vi "Periodic Tasks.vi"(8 "error in":errorcluster) -> ()   [LabVIEW 2015]
doc: "This VI runs in parallel to other tasks. It can contain as many user-defined periodic loops as you need. These can carry out PID or other sorts of timed response."
uses:
  <vilib>/Rock Robotics/WPI/Utilities/WPI_GetSetVariantRefNum.vi
  Robot Global Data.vi
  <vilib>/Rock Robotics/Network Tables/SD Write Number.vi
  <vilib>/Rock Robotics/Network Tables/SD Write Boolean.vi
  <vilib>/Rock Robotics/Network Tables/NT Read Numeric Array.vi
  <vilib>/Rock Robotics/Network Tables/SD Write Numeric Array.vi
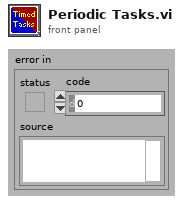
[diagram p1: front panel]
types:
  T1 = typedef "WPI_JoystickDevRef.ctl" = cluster{"Device":T2}
  T2 = typedef "WPI_JoystickDeviceEnum.ctl" = enum16{"USB 0", "USB 1", "USB 2", "USB 3", "USB 4", "USB 5"}
  T3 = cluster{"Axes[0]":dbl, "Axes[1]":dbl, "Axes[2]":dbl, "Axes[3]":dbl, "Axes[4]":dbl, "Axes[5]":dbl, "Axes[6]":dbl, "Axes[7]":dbl, "Axes[8]":dbl}
  T4 = cluster{"Buttons[0]":bool, "Buttons[1]":bool, "Buttons[2]":bool, "Buttons[3]":bool, "Buttons[4]":bool, "Buttons[5]":bool, "Buttons[6]":bool, "Buttons[7]":bool, "Buttons[8]":bool}
  T5 = typedef "WPI_EncoderDevRef.ctl" = cluster{"DevStatus":errorcluster, "EncoderIndex":T6, "CounterIndex":T7, "DistancePerCount":dbl, "Decoding Type":T8}
  T6 = typedef "FPGA_EncoderIdx.ctl" = enum8{"Enc 0", "Enc 1", "Enc 2", "Enc 3", "Enc 4", "Enc 5", "Enc 6", "Enc 7", "Invalid"}
  T7 = typedef "FPGA_CounterCtrSystemIndex.ctl" = enum8{"Ctr 0", "Ctr 1", "Ctr 2", "Ctr 3", "Ctr 4", "Ctr 5", "Ctr 6", "Ctr 7", "Invalid"}
  T8 = typedef "WPI_EncoderType.ctl" = enum16{"1x", "2x", "4x"}
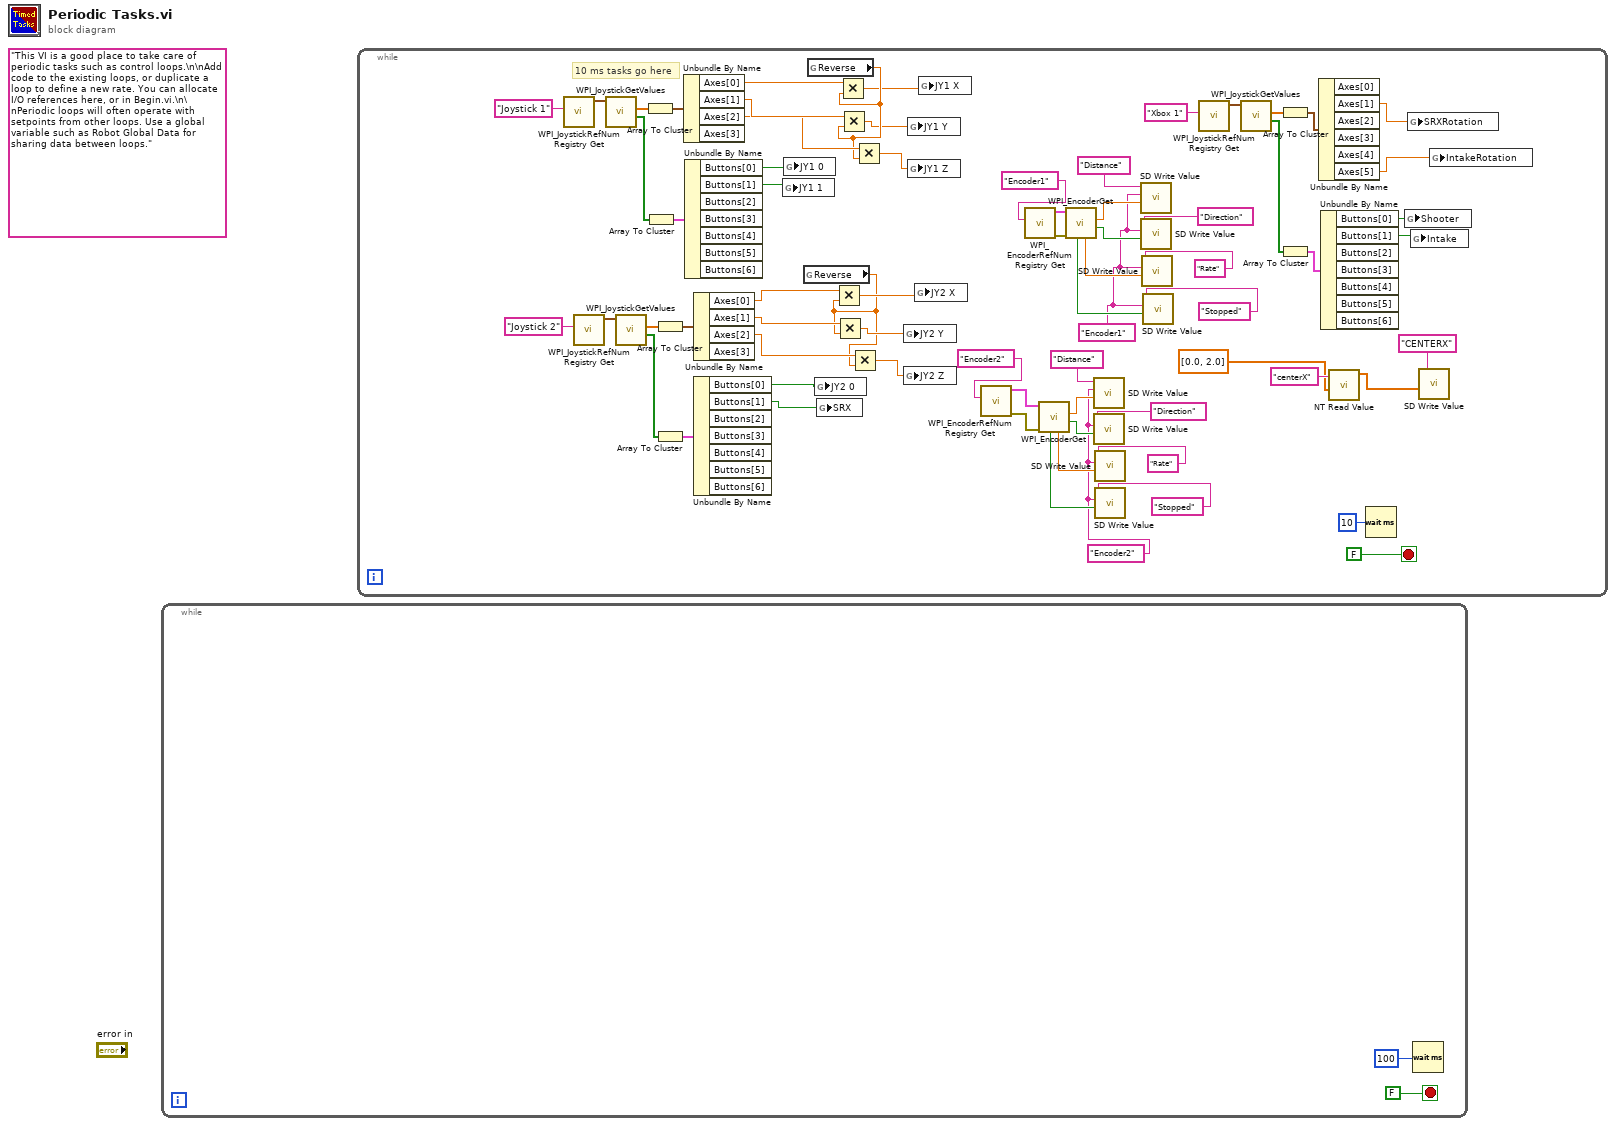
[diagram p0: block diagram]
diagram:
  (unwired) "This VI is a good place to take care of periodic tasks such as control loops.\n\nAdd code to the existing loops, or duplicate a loop to define a new rate. You can allocate I/O references here, or in Begin.vi.\n\nPeriodic loops will often operate with setpoints from other loops. Use a global variable such as Robot Global Data for sharing data between loops."
  n1 = while {
    stop <- FALSE stop-if-true
    n2 = Wait (ms)(milliseconds to wait=u32 100) -> ()  [unwired: 1 out]
  }
  n3 = while {
    stop <- FALSE stop-if-true
    w11 = "Encoder2"
    w10 = "Encoder1"
    # "10 ms tasks go here"
    n4 = call <vilib>:"WPI_JoystickRefNum Registry Get.vi"("refnum name"="Joystick 1") -> ("JoystickDevRef"=w71:T1)  [unwired: 1 in, 9 out]
    n5 = call <vilib>:"WPI_JoystickRefNum Registry Get.vi"("refnum name"="Joystick 2") -> ("JoystickDevRef"=w65:T1)  [unwired: 1 in, 9 out]
    n6 = call <vilib>:"WPI_JoystickGetValues.vi"("JoystickDevRef"=w71) -> ("Buttons"=w69:bool[], "Axes"=w68:dbl[])  [unwired: 6 in, 3 out]
    n7 = call <vilib>:"WPI_JoystickGetValues.vi"("JoystickDevRef"=w65) -> ("Buttons"=w63:bool[], "Axes"=w62:dbl[])  [unwired: 6 in, 3 out]
    n8 = Array To Cluster(array=w68) -> (cluster=w70:T3)
    n9 = Array To Cluster(array=w69) -> (cluster=w67:T4)
    n10 = Array To Cluster(array=w62) -> (cluster=w64:T3)
    n11 = Array To Cluster(array=w63) -> (cluster=w61:T4)
    n12 = Unbundle By Name(w70) -> ("Axes[0]"=w58:dbl, "Axes[1]"=w57:dbl, "Axes[2]"=w56:dbl)  [unwired: 1 out]
    n13 = Unbundle By Name(w67) -> ("Buttons[0]"=w60:bool, "Buttons[1]"=w59:bool)  [unwired: 5 out]
    n14 = Unbundle By Name(w64) -> ("Axes[0]"=w48:dbl, "Axes[1]"=w47:dbl, "Axes[2]"=w46:dbl)  [unwired: 1 out]
    n15 = Unbundle By Name(w61) -> ("Buttons[0]"=w44:bool, "Buttons[1]"=w30:bool)  [unwired: 5 out]
    n16 = global write "Robot Global Data.vi" "JY1 1"(w59) -> ()
    n17 = global write "Robot Global Data.vi" "JY1 0"(w60) -> ()
    n18 = global read "Robot Global Data.vi" "Reverse"() -> (w45:dbl)
    n19 = global read "Robot Global Data.vi" "Reverse"() -> (w55:dbl)
    n20 = global write "Robot Global Data.vi" "JY2 0"(w44) -> ()
    n21 = global write "Robot Global Data.vi" "SRX"(w30) -> ()
    n22 = Multiply(x=w48, y=w45) -> (x*y=w51:dbl)
    n23 = Multiply(x=w47, y=w45) -> (x*y=w50:dbl)
    n24 = Multiply(x=w58, y=w55) -> (x*y=w54:dbl)
    n25 = Multiply(x=w57, y=w55) -> (x*y=w53:dbl)
    n26 = Multiply(x=w46, y=w45) -> (x*y=w49:dbl)
    n27 = Multiply(x=w56, y=w55) -> (x*y=w52:dbl)
    n28 = global write "Robot Global Data.vi" "JY2 Y"(w50) -> ()
    n29 = global write "Robot Global Data.vi" "JY2 Z"(w49) -> ()
    n30 = global write "Robot Global Data.vi" "JY1 Y"(w53) -> ()
    n31 = global write "Robot Global Data.vi" "JY1 Z"(w52) -> ()
    n32 = global write "Robot Global Data.vi" "JY2 X"(w51) -> ()
    n33 = global write "Robot Global Data.vi" "JY1 X"(w54) -> ()
    n34 = call <vilib>:"WPI_EncoderRefNum Registry Get.vi"("refnum name"="Encoder2") -> ("error out"=w22:errorcluster, "EncoderDevRef"=w21:T5)  [unwired: 9 in]
    n35 = call <vilib>:"WPI_EncoderRefNum Registry Get.vi"("refnum name"="Encoder1") -> ("error out"=w43:errorcluster, "EncoderDevRef"=w42:T5)  [unwired: 9 in]
    n36 = call <vilib>:"WPI_EncoderGet.vi"("error in (no error)"=w22, "EncoderDevRef"=w21) -> ("Direction"=w18:bool, "Distance"=w19:dbl, "Rate"=w17:dbl, "Stopped"=w16:bool)  [unwired: 4 in, 2 out]
    n37 = call <vilib>:"WPI_EncoderGet.vi"("error in (no error)"=w43, "EncoderDevRef"=w42) -> ("Direction"=w39:bool, "Distance"=w40:dbl, "Rate"=w38:dbl, "Stopped"=w37:bool)  [unwired: 4 in, 2 out]
    n38 = call-poly <vilib>:"SD Write Value.vi"("Numeric"=w19, "Table Prefix"=w11, "Name"="Distance") -> ()  [unwired: 7 in, 2 out]
    n39 = call-poly <vilib>:"SD Write Value.vi"("Boolean"=w18, "Table Prefix"=w11, "Name"="Direction") -> ()  [unwired: 7 in, 2 out]
    n40 = call-poly <vilib>:"SD Write Value.vi"("Numeric"=w17, "Table Prefix"=w11, "Name"="Rate") -> ()  [unwired: 7 in, 2 out]
    n41 = call-poly <vilib>:"SD Write Value.vi"("Boolean"=w16, "Table Prefix"=w11, "Name"="Stopped") -> ()  [unwired: 7 in, 2 out]
    n42 = call-poly <vilib>:"SD Write Value.vi"("Numeric"=w40, "Table Prefix"=w10, "Name"="Distance") -> ()  [unwired: 7 in, 2 out]
    n43 = call-poly <vilib>:"SD Write Value.vi"("Boolean"=w39, "Table Prefix"=w10, "Name"="Direction") -> ()  [unwired: 7 in, 2 out]
    n44 = call-poly <vilib>:"SD Write Value.vi"("Numeric"=w38, "Table Prefix"=w10, "Name"="Rate") -> ()  [unwired: 7 in, 2 out]
    n45 = call-poly <vilib>:"SD Write Value.vi"("Boolean"=w37, "Table Prefix"=w10, "Name"="Stopped") -> ()  [unwired: 7 in, 2 out]
    n46 = call <vilib>:"WPI_JoystickRefNum Registry Get.vi"("refnum name"="Xbox 1") -> ("JoystickDevRef"=w28:T1)  [unwired: 1 in, 9 out]
    n47 = call <vilib>:"WPI_JoystickGetValues.vi"("JoystickDevRef"=w28) -> ("Buttons"=w26:bool[], "Axes"=w25:dbl[])  [unwired: 6 in, 3 out]
    n48 = Array To Cluster(array=w25) -> (cluster=w27:T3)
    n49 = Array To Cluster(array=w26) -> (cluster=w24:T4)
    n50 = Unbundle By Name(w27) -> ("Axes[1]"=w5:dbl, "Axes[5]"=w4:dbl)  [unwired: 4 out]
    n51 = Unbundle By Name(w24) -> ("Buttons[0]"=w23:bool, "Buttons[1]"=w3:bool)  [unwired: 5 out]
    n52 = call-poly <vilib>:"NT Read Value.vi"("Default Value"=dbl[] [0.0, 2.0], "Name"="centerX") -> ("Numeric Array"=w8:dbl[])  [unwired: 8 in, 1 out]
    n53 = Wait (ms)(milliseconds to wait=u32 10) -> ()  [unwired: 1 out]
    n54 = global write "Robot Global Data.vi" "Shooter"(w23) -> ()
    n55 = global write "Robot Global Data.vi" "SRXRotation"(w5) -> ()
    n56 = global write "Robot Global Data.vi" "Intake"(w3) -> ()
    n57 = call-poly <vilib>:"SD Write Value.vi"("Numeric Array"=w8, "Name"="CENTERX") -> ()  [unwired: 8 in, 2 out]
    n58 = global write "Robot Global Data.vi" "IntakeRotation"(w4) -> ()
  }
